vi "Cell I Readback.vi"(7 "Box ID":u8, 8 "error in (no error)":errorcluster, 10 "Channel":u16=1 min=1 max=12 step=1, 11 "ENET in":refnum<class "ENET_BS120x.lvclass">) -> (0 "error out":errorcluster, 2 "Current (mA)":dbl, 3 "ENET out":refnum<class "ENET_BS120x.lvclass">)   [LabVIEW 2021, in "BS120x Driver.lvlib" / "ENET_BS120x.lvclass"]
uses:
  ENET_BS120x.lvclass
  BS120x.lvclass
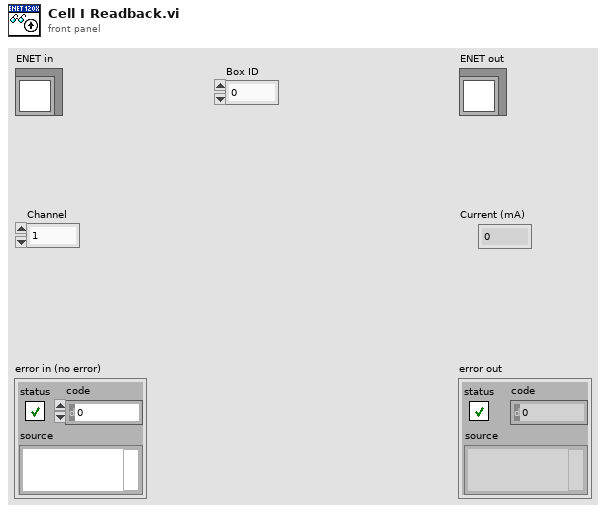
[diagram p1: front panel]
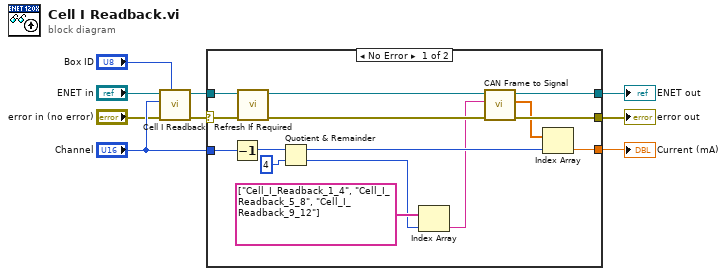
[diagram p0: block diagram]
diagram:
  n1 = call-parent "Cell I Readback.vi"("Box ID"="Box ID", "error in (no error)"="error in (no error)", "Channel"="Channel", "BS120x in"="ENET in") -> ("error out"=w2:errorcluster, "BS120x out"=w5:refnum<class "ENET_BS120x.lvclass">)  [unwired: 5 in, 1 out]
  n2 = case shown="No Error" w2 {
    selector: w2 -> [w13 w25]
    tunnel: [w24 w25] -> w9
    tunnel: [w19 _] -> w8
    tunnel: [w18 w26] -> w7
    tunnel: w5 -> [w15 w26]
    tunnel: "Channel" -> [w14 _]
    frame No Error {
      n3 = Decrement(x=w14) -> (x-1=w22:u16)
      n4 = call "Refresh If Required.vi"("error in (no error)"=w13, "Ethernet in"=w15) -> ("error out"=w17:errorcluster, "Ethernet out"=w16:refnum<class "ENET_BS120x.lvclass">)  [unwired: 8 in]
      n5 = Quotient & Remainder(x=w22, y=u16 4) -> (x-y*floor(x/y)=w21:u16, floor(x/y)=w11:u16)
      n6 = Index Array(array=string[] ["Cell_I_Readback_1_4", "Cell_I_Readback_5_8", "Cell_I_Readback_9_12"], index=w11) -> (element=w10:string)
      n7 = call "CAN Frame to Signal.vi"("error in (no error)"=w17, "Frame"=w10, "ENET in"=w16) -> ("error out"=w24:errorcluster, "signal data"=w20:dbl[], "ENET out"=w18:refnum<class "ENET_BS120x.lvclass">)  [unwired: 6 in]
      n8 = Index Array(array=w20, index=w21) -> (element=w19:dbl)
    }
    frame Error {
    }
  }
  "error out" <- w9
  "ENET out" <- w7
  "Current (mA)" <- w8
